vi "Set_Do_Array.vi"(8 "error in (no error)":errorcluster, 10 "DOs":bool[](array[boolean]), 11 "reference in":refnum<class "FPGA_Concrete.lvclass">) -> (0 "error out":errorcluster, 3 "reference out":refnum<class "FPGA_Concrete.lvclass">)   [LabVIEW 2019, in "FPGA_Concrete.lvclass"]
uses:
  FPGA_Concrete.lvclass
  FPGA_Concrete.lvclass/FPGA_Concrete.ctl
  <vilib>/Utility/error.llb/Error Cluster From Error Code.vi
  <vilib>/rvi/errors/niLvFpgaAdjustHostInterfaceError.vi
  <vilib>/rvi/interface/nirviReadWriteControl/nirviReadWriteControl.xnode
  FPGA VI Reference.ctl
  NiFpgaLv.dll
  <vilib>/rvi/interface/Simulation/niFpgaSimulationCallBeginRW.vi
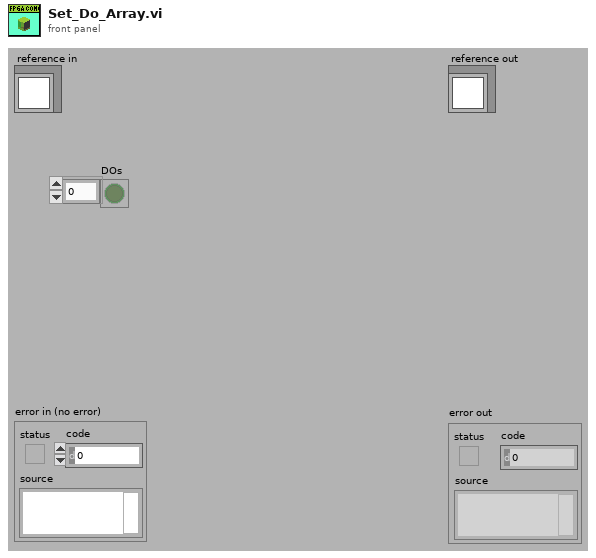
[diagram p1: front panel]
types:
  T1 = typedef "FPGA_Concrete.lvclass/FPGA VI Reference.ctl" = refnum<k20>
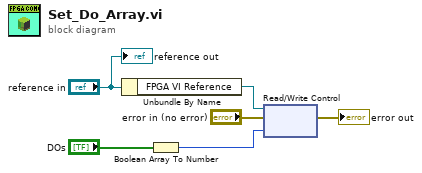
[diagram p0: block diagram]
diagram:
  n1 = Unbundle By Name("reference in") -> ("FPGA VI Reference"=w6:T1)
  n2 = Boolean Array To Number(Boolean array="DOs") -> (number=w3:u32)
  n3 = xnode "Read/Write Control"("FPGA VI Reference In"=w6, "error in"="error in (no error)", "DOs"=w3) -> ("error out"=→"error out":errorcluster)  [unwired: 1 out]
  "reference out" <- "reference in"
